vi "Digital Command.vi"(8 "error in (no error)":errorcluster, 9 "CmdDigital":T1, 11 "ValveControlModule in":refnum<class "DigitalControlModule.lvclass">) -> (0 "error out":errorcluster, 3 "ValveControlModule out":refnum<class "DigitalControlModule.lvclass">)   [LabVIEW 2020, in "VolatusControl.lvlib" / "DigitalControlModule.lvclass"]
uses:
  DigitalControlModule.lvclass
  DigitalControlModule.lvclass/DigitalControlModule.ctl
  DigitalControl/DigitalControl.lvclass
  messages/CmdDigital/Data.ctl
  messages/CmdDigital/CmdDigital.lvlib
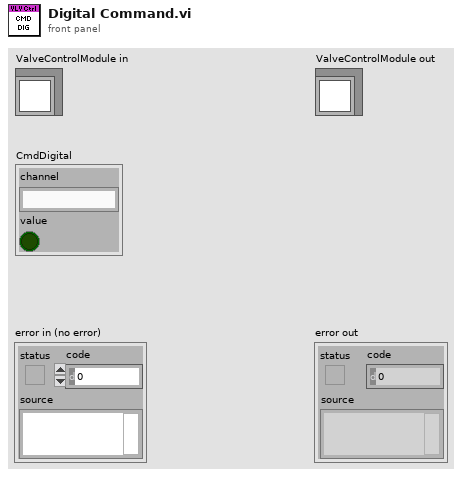
[diagram p1: front panel]
types:
  T1 = typedef "CmdDigital.lvlib/Data.ctl" = cluster{"channel":string, "value":bool}
  T2 = map{string, refnum<class "DigitalControl.lvclass">}
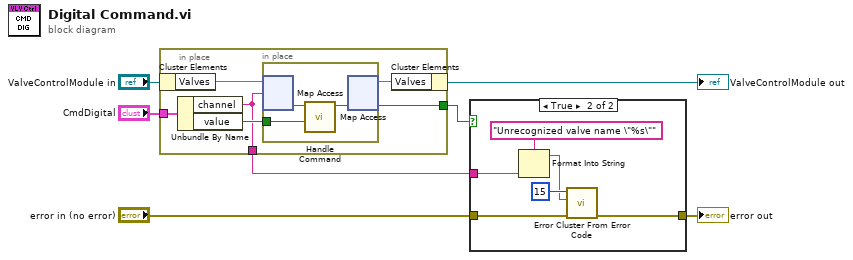
[diagram p0: block diagram]
diagram:
  n1 = in-place {
    in-place-border: "CmdDigital" -> [w13]
    in-place-border: [w9] -> w7
    in-place-border: [w8] -> w6
    n2 = in-place-cluster #1("ValveControlModule in") -> ("Valves"=w12:T2)
    n3 = Unbundle By Name(w13) -> ("channel"=w8:string, "value"=w11:bool)
    n4 = in-place {
      in-place-border: w11 -> [w15]
      n5 = in-place-map #2(w12, w8) -> (w16:refnum<class "DigitalControl.lvclass">)  [unwired: 1 in, 1 out]
      n6 = call-dynamic "Handle Command.vi"("Value"=w15, "Valve in"=w16) -> ("Valve out"=w14:refnum<class "DigitalControl.lvclass">)  [unwired: 8 in, 1 out]
      n7 = in-place-map #2(w14) -> (w10:T2, w9:bool)  [unwired: 1 in, 1 out]
    }
    n8 = in-place-cluster #1("Valves"=w10) -> (→"ValveControlModule out":refnum<class "DigitalControlModule.lvclass">)
  }
  n9 = case shown="True" w7 {
    tunnel: w6 -> [_ w23]
    tunnel: "error in (no error)" -> [w17 w19]
    tunnel: [w17 w18] -> w3
    frame False {
    }
    frame True {
      n10 = Format Into String(format string="Unrecognized valve name \"%s\"", w23) -> (resulting string=w20:string)  [unwired: 2 in, 1 out]
      n11 = call <vilib>:"Error Cluster From Error Code.vi"("error in (no error)"=w19, "error message (\"\")"=w20, "error code (0)"=15) -> ("error out"=w18:errorcluster)  [unwired: 6 in]
    }
  }
  "error out" <- w3
